vi "initialize buffer.vi"(0 "Periode":i64, 5 "samplesize plots":i64=600, 9 "initial time":dbl) -> (8 "buffer plot":cluster{"X":dbl[], "Y":dbl[]})   [LabVIEW 2010]
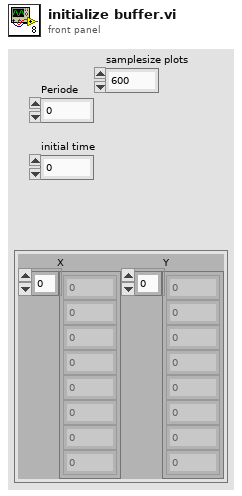
[diagram p1: front panel]
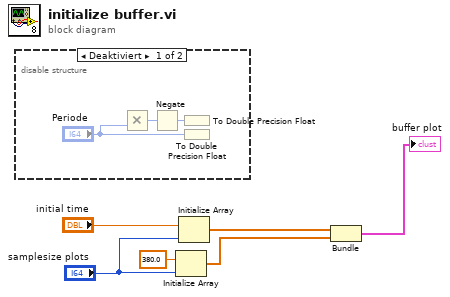
[diagram p0: block diagram]
diagram:
  n1 = disable-structure shown="Deaktiviert" {
    frame Disabled {
      n2 = Multiply(y="Periode") -> (x*y=w8:i64)  [unwired: 1 in]
      n3 = Negate(x=w8) -> (-x=w9:i64)
      n4 = To Double Precision Float(number=w9) -> ()  [unwired: 1 out]
      n5 = To Double Precision Float(number="Periode") -> ()  [unwired: 1 out]
    }
    frame Enabled {
    }
  }
  n6 = Initialize Array(380.0 ("Element"), "samplesize plots") -> (w2:dbl[])
  n7 = Initialize Array("initial time", "samplesize plots") -> (w4:dbl[])
  n8 = Bundle(w4, w2) -> (→"buffer plot":cluster{dbl[], dbl[]})  [unwired: 1 in]
